vi "SetCellValueByString.vi"(4 "As Number":bool=TRUE, 6 "Value":string, 7 "WorkSheetName":string, 8 "error in (no error)":errorcluster, 9 "Column Index":i32, 10 "Row Index":i32, 11 "ExcelFile in":refnum<class "PortableExcelFileManipulationOXML.lvclass">) -> (0 "error out":errorcluster, 3 "ExcelFile out":refnum<class "PortableExcelFileManipulationOXML.lvclass">)   [LabVIEW 2019, in "PortableExcelFileManipulationOXML.lvclass"]
doc: "Sets A Cell value on an excel spreadsheet, The inputs allow the value to be input as string or a number. It also allows the worksheet index to be chosen."
uses:
  PortableExcelFileManipulationOXML.lvclass
  PortableExcelFileManipulationOXML.lvclass/PortableExcelFileManipulationOXML.ctl
  H:/LV projects/ExpressionEvaluator/Excel/ExcelManipulation.dll
  ExcelManipulation.dll
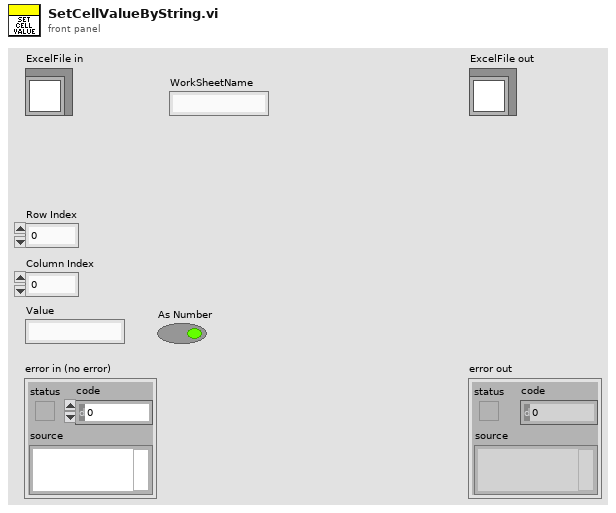
[diagram p1: front panel]
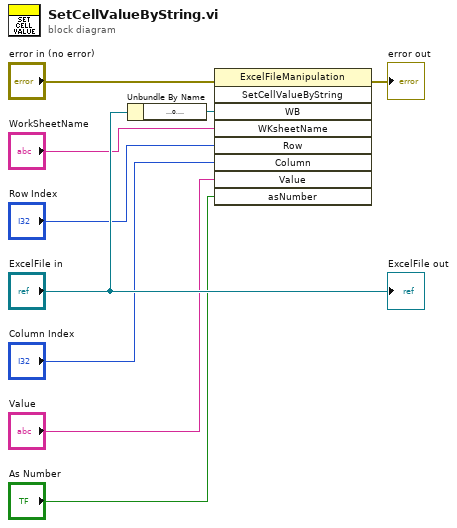
[diagram p0: block diagram]
diagram:
  n1 = Unbundle By Name("ExcelFile in") -> ("ExcelOpen"=w8:refnum<k24>)
  n2 = invoke class="ExcelFileManipulation" method="SetCellValueByString"(error in="error in (no error)", "WB"=w8, "WKsheetName"="WorkSheetName", "Row"="Row Index", "Column"="Column Index", "Value"="Value", "asNumber"="As Number") -> (error out=→"error out":errorcluster)  [unwired: 2 in, 8 out]
  "ExcelFile out" <- "ExcelFile in"
